vi "Agilent VNA Read Error Message Mode.vi"(7 "Agilent VNA":T1, 8 "error in (no error)":errorcluster, 11 "VISA Resource Name":refnum<visa-resource-name>) -> (0 "error out":errorcluster, 2 "Error Message Mode":T2=enum."Off", 3 "dup VISA Resource Name":refnum<visa-resource-name>)   [LabVIEW 2011]
doc: "This VI for the HP8753B Network Analyzers reads the stimulus values. Except when performing log sweeps and freq list sweeps, this VI uses the start and stop values and the number of points to calcuate the stimulus values."
uses:
  TypeDefs/Agilent VNA Error Message Mode.ctl
  TypeDefs/Agilent VNA Instrument Info.ctl
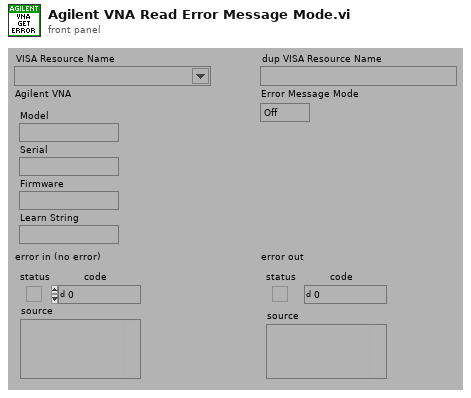
[diagram p1: front panel]
types:
  T1 = typedef "Agilent VNA Instrument Info.ctl" = cluster{"Model":string, "Serial":string, "Firmware":string, "Learn String":string}
  T2 = typedef "Agilent VNA Error Message Mode.ctl" = enum16{"On", "Off"}
  T3 = typedef "Agilent VNA Model.ctl" = enum16{"Not Supported", "8510X", "8719X", "8720X", "8722X", "8753X", "ENA", "PNA", "Field Fox"}
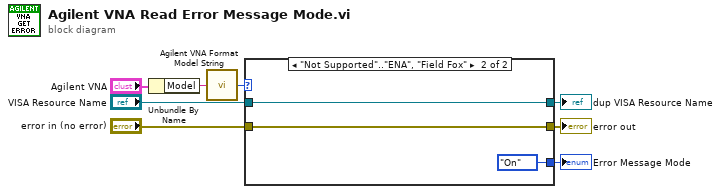
[diagram p0: block diagram]
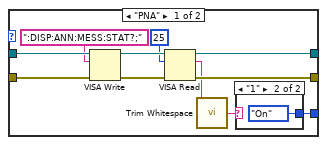
[diagram p2: hidden frame]
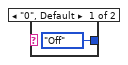
[diagram p3: hidden frame]
diagram:
  n1 = Unbundle By Name("Agilent VNA") -> ("Model"=w1:string)
  n2 = call "Agilent VNA Format Model String.vi"("Model"=w1) -> ("Model"=w3:T3)
  n3 = case shown="\"Not Supported\"..\"ENA\", \"Field Fox\"" w3 {
    tunnel: "error in (no error)" -> [w15 w23]
    tunnel: [w14 w23] -> w7
    tunnel: "VISA Resource Name" -> [w16 w24]
    tunnel: [w13 w24] -> w5
    tunnel: [w9 Agilent_VNA_Error_Message_Mode."On"] -> w4
    frame "PNA" {
      n4 = VISA Write(VISA resource name=w16, write buffer=":DISP:ANN:MESS:STAT?;", error in (no error)=w15) -> (VISA resource name out=w19:refnum<visa-resource-name>, error out=w18:errorcluster)  [unwired: 1 out]
      n5 = VISA Read(VISA resource name=w19, byte count=u32 25, error in (no error)=w18) -> (VISA resource name out=w13:refnum<visa-resource-name>, read buffer=w11:string, error out=w14:errorcluster)  [unwired: 1 out]
      n6 = call <vilib>:"Trim Whitespace.vi"("string"=w11) -> ("trimmed string"=w10:string)  [unwired: 1 in]
      n7 = case shown="\"1\"" w10 {
        tunnel: [Agilent_VNA_Error_Message_Mode."Off" Agilent_VNA_Error_Message_Mode."On"] -> w9
        frame "0", Default {
        }
        frame "1" {
        }
      }
    }
    frame "Not Supported".."ENA", "Field Fox" {
    }
  }
  "dup VISA Resource Name" <- w5
  "error out" <- w7
  "Error Message Mode" <- w4
